vi "Pose2d to Rigid Transform.vi"(11 "Pose2d":T1) -> (3 "Rigid Transform":T4)   [LabVIEW 2019]
uses:
  <vilib>/Analysis/Matrix/Datatypes/RealMatrix.ctl
  Typedef/Pose2d.ctl
  Typedef/Translation2d.ctl
  Typedef/Rotation2d.ctl
  <vilib>/Analysis/Matrix/NI_Matrix.lvlib
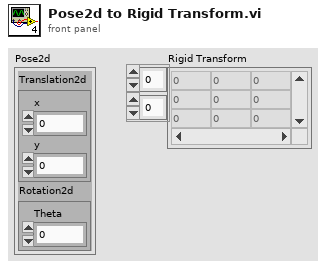
[diagram p1: front panel]
types:
  T1 = typedef "Pose2d.ctl" = cluster{"Translation2d":T2, "Rotation2d":T3}
  T2 = typedef "Translation2d.ctl" = cluster{"x":dbl, "y":dbl}
  T3 = typedef "Rotation2d.ctl" = cluster{"Theta":dbl}
  T4 = typedef "NI_Matrix.lvlib/RealMatrix.ctl" = dbl[][]
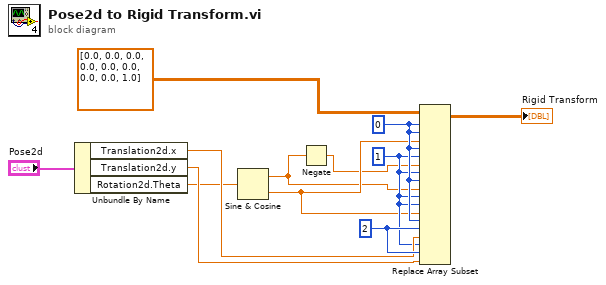
[diagram p0: block diagram]
diagram:
  w10 = 2 ("index (col)")
  w7 = 1 ("disabled index (col)")
  w8 = 0 ("disabled index (row)")
  n1 = Unbundle By Name("Pose2d") -> ("Translation2d.x"=w9:dbl, "Translation2d.y"=w11:dbl, "Rotation2d.Theta"=w2:dbl)
  n2 = Sine & Cosine(0:w2) -> (1:w5:dbl, 2:w6:dbl)
  n3 = Negate(x=w5) -> (-x=w4:dbl)
  n4 = Replace Array Subset(array=T4 [[0.0, 0.0, 0.0], [0.0, 0.0, 0.0], [0.0, 0.0, 1.0]] ("appended array"), new element #1=w6, index (row) #1=w8, index (col) #1=w8, new element #2=w4, index (row) #2=w8, index (col) #2=w7, new element #3=w5, index (row) #3=w7, index (col) #3=w8, new element #4=w6, index (row) #4=w7, index (col) #4=w7, new element #5=w9, index (row) #5=w8, index (col) #5=w10, new element #6=w11, index (row) #6=w7, index (col) #6=w10) -> (→"Rigid Transform":T4)
